vi "Export XY Graph Image to Notebook.vi"(8 "Error In":errorcluster, 9 "XYGraph Ref":refnum<vi>, 11 "Notebook Q":refnum<queue>) -> (0 "Error Out":errorcluster)   [LabVIEW 2019, in "Notebook.lvlib"]
uses:
  Notebook.lvlib
  Notebook Action Q Element.ctl
  Notebook Action List.ctl
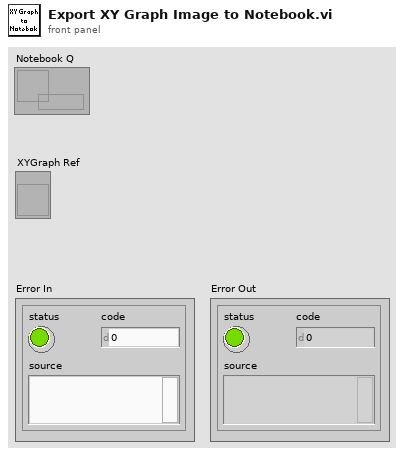
[diagram p1: front panel]
types:
  T1 = typedef "Notebook.lvlib/Notebook Action Q Element.ctl" = cluster{"Action":T2, "Variant":variant}
  T2 = typedef "Notebook.lvlib/Notebook Action List.ctl" = enum16{"Idle", "Init", "Check Content Change", "User added content", "Program added text", "Program added Picture ", "Save Notebook", "Quit", "Open", "Close", "Update Window Title"}
  T3 = typedef "imagedata.ctl" = cluster{"image type":i32, "image depth":i32, "image":u8[], "mask":u8[], "colors":u32[], "Rectangle":cluster{"left":i16, "top":i16, "right":i16, "bottom":i16}}
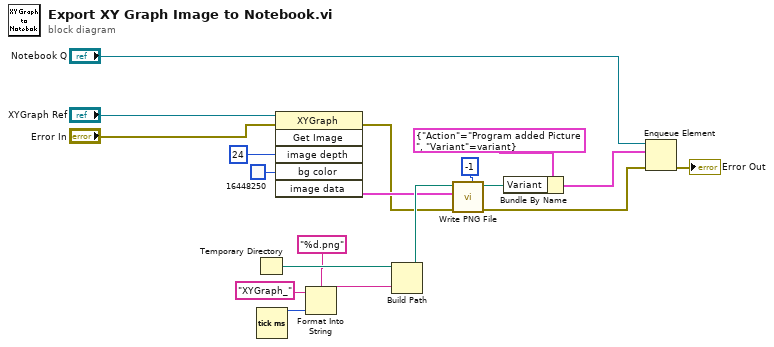
[diagram p0: block diagram]
diagram:
  n1 = Temporary Directory() -> (w14:path)
  n2 = Tick Count (ms)() -> (millisecond timer value=w13:u32)
  n3 = invoke on="Invoke Node" class="XYGraph" method="Get Image"(reference="XYGraph Ref", error in="Error In", "image depth"=24 ("Image Depth"), "bg color"=u32 16448250) -> (error out=w3:errorcluster, "image data"=w8:T3)  [unwired: 2 in, 4 out]
  n4 = Format Into String(format string="%d.png", initial string="XYGraph_", w13) -> (resulting string=w12:string)  [unwired: 1 in, 1 out]
  n5 = Build Path(base path=w14, name or relative path=w12) -> (appended path=w9:path)
  n6 = call <vilib>:"Write PNG File.vi"("compression (default)"=-1, "error in (no error)"=w3, "image data"=w8, "path to PNG file"=w9) -> ("error out"=w2:errorcluster, "path"=w7:path)  [unwired: 6 in]
  n7 = Bundle By Name(cluster=T1 {"Action"=enum."Program added Picture ", "Variant"=variant} ("element"), "Variant"=w7) -> (w5:T1)
  n8 = Enqueue Element(queue="Notebook Q", element=w5, error in (no error)=w2) -> (error out=→"Error Out":errorcluster)  [unwired: 1 in, 2 out]
